vi "green_buoy_thresholding1.0.vi"(4 "Cluster":cluster{"Min Radius":sgl, "Max Radius":sgl}={"Min Radius"=3.0, "Max Radius"=100.0}, 5 "Blue or Luma or Val or Inten Range":cluster{"Lower value":i32, "Upper value":i32}={"Lower value"=0, "Upper value"=255}, 7 "error in (no error)":errorcluster, 8 "Green or Sat Range":cluster{"Lower value":i32, "Upper value":i32}={"Lower value"=0, "Upper value"=255}, 9 "Red or Hue Range":cluster{"Lower value":i32, "Upper value":i32}={"Lower value"=50, "Upper value"=102}, 10 "Image Src":T2) -> (0 "error out":errorcluster, 1 "Circles Data (calibrated)":T1(array[cluster]), 2 "Nb Circles":i32, 3 "Image Out":T2(plugin-control))   [LabVIEW 2009]
uses:
  <vilib>/vision/Image Controls.llb/IMAQ Image.ctl
  <vilib>/vision/NI_Vision_Development_Module.lvlib
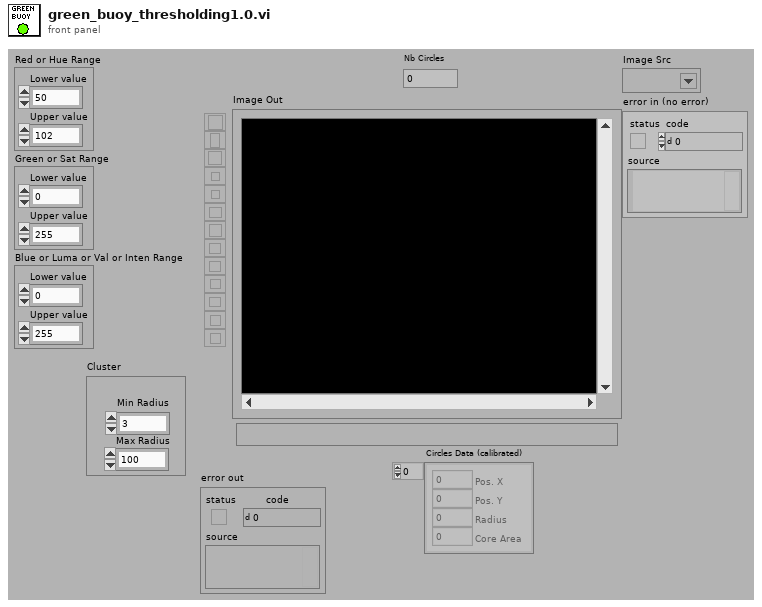
[diagram p1: front panel]
types:
  T1 = cluster{"Pos. X":i32, "Pos. Y":i32, "Radius":i32, "Core Area":i32}[]
  T2 = typedef "IMAQ Image.ctl" = refnum<image>
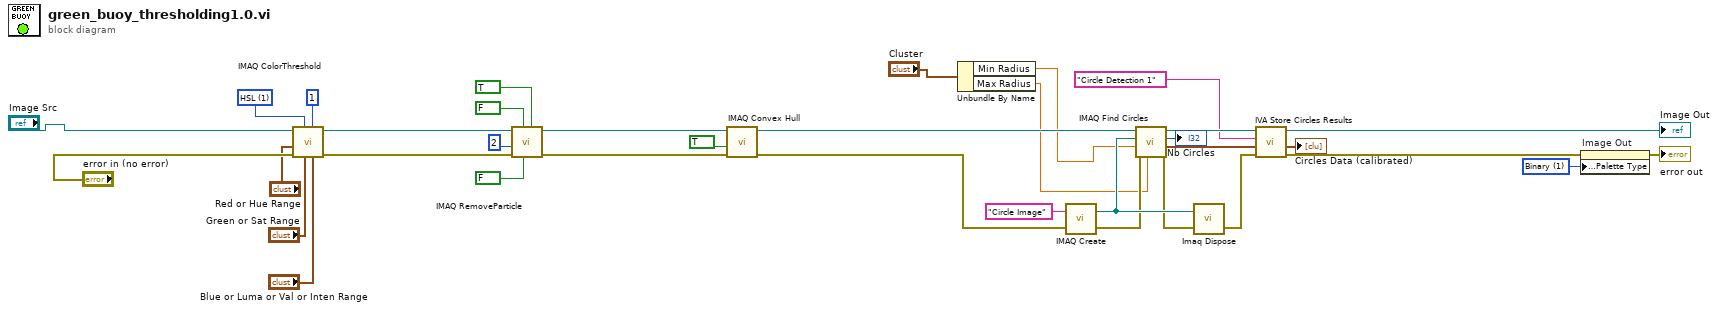
[diagram p0: block diagram]
diagram:
  w8 = u32 1 items=["Grayscale", "Binary", "Gradient", "Rainbow", "Temperature", "User Defined"] ("Palette")
  w32 = u16 1 items=["RGB", "HSL", "HSV", "HSI"] ("Color Mode")
  n1 = call "IMAQ ColorThreshold"("Blue or Luma or Val or Inten Range"="Blue or Luma or Val or Inten Range", "Replace Value"=1, "Green or Sat Range"="Green or Sat Range", "Color Mode"=w32, "error in (no error)"="error in (no error)", "Red or Hue Range"="Red or Hue Range", "Image Src"="Image Src") -> ("error out"=w28:errorcluster, "Image Dst Out"=w23:T2)  [unwired: 1 in, 2 out]
  n2 = call "IMAQ RemoveParticle"("Connectivity 4/8 (8)"=TRUE, "Low Pass/High Pass (Low)"=FALSE, "Square/Hexa (Square)"=FALSE, "error in (no error)"=w28, "Number of Erosion"=2, "Image Src"=w23) -> ("error out"=w22:errorcluster, "Image Dst Out"=w21:T2)  [unwired: 1 in, 3 out]
  n3 = call "IMAQ Convex Hull"("error in (no error)"=w22, "Connectivity 4/8 (8)"=TRUE, "Image Src"=w21) -> ("error out"=w19:errorcluster, "Image Dst Out"=w12:T2)  [unwired: 1 in, 6 out]
  n4 = Unbundle By Name("Cluster") -> ("Min Radius"=w3:sgl, "Max Radius"=w4:sgl)
  n5 = call "IMAQ Create"("Image Name"="Circle Image", "error in (no error)"=w19) -> ("New Image"=w17:T2, "error out"=w16:errorcluster)  [unwired: 2 in, 1 out]
  n6 = call "IMAQ Find Circles"("Max Radius"=w4, "error in (no error)"=w16, "Min Radius"=w3, "Image Dst"=w17, "Image Src"=w12) -> ("error out"=w15:errorcluster, "Circles Data"=w10:T1, "Nb Circles"=→"Nb Circles":i32)  [unwired: 4 out]
  n7 = call "Imaq Dispose"("Image"=w17, "error in (no error)"=w15) -> ("error out"=w14:errorcluster)  [unwired: 1 in, 3 out]
  n8 = call <vilib>:"IVA Store Circles Results.vi"("error in (no error)"=w14, "Circles Data"=w10, "Step Name"="Circle Detection 1", "Image in"=w12) -> ("error out"=w13:errorcluster, "Circles Data (calibrated)"=→"Circles Data (calibrated)":T1, "Image dup"=→"Image Out":T2)  [unwired: 5 out]
  n9 = property on="Image Out" class="ImageControl"(error in=w13, "Palette:Palette Type"=w8) -> (error out=→"error out":errorcluster)  [unwired: 1 in, 1 out]
